vi "Update Filter.vi"(8 "error in (no error)":errorcluster, 10 "Filter in":refnum<class "Filter.lvclass">, 11 "Debugger in":refnum<class "Debugger.lvclass">) -> (0 "error out":errorcluster, 3 "Debugger out":refnum<class "Debugger.lvclass">)   [LabVIEW 2020, in "Debugger.lvclass"]
uses:
  Debugger.lvclass
  Filter/Filter.lvclass
  Debugger.lvclass/Debugger.ctl
  Debug Log/Debug Log.lvclass
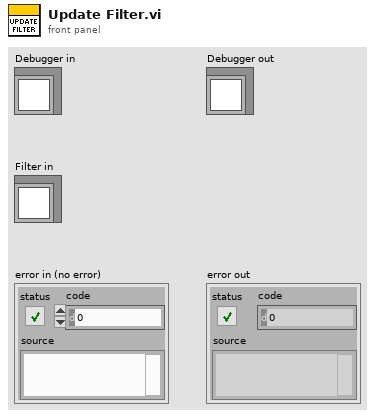
[diagram p1: front panel]
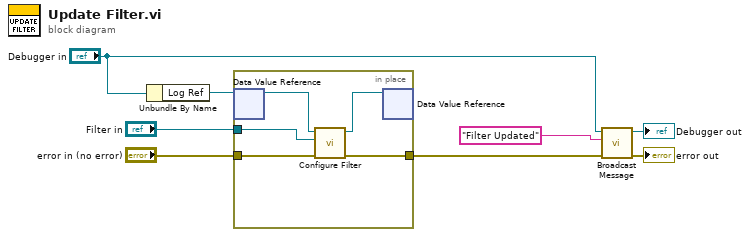
[diagram p0: block diagram]
diagram:
  n1 = Unbundle By Name("Debugger in") -> ("Log Ref"=w1:refnum<data-value>)
  n2 = in-place {
    in-place-border: "error in (no error)" -> [w13]
    in-place-border: "Filter in" -> [w12]
    in-place-border: [w11] -> w6
    n3 = in-place-dvr #1(w1) -> (w10:refnum<class "Debug Log.lvclass">)  [unwired: 1 out]
    n4 = call "Configure Filter.vi"("error in (no error)"=w13, "Filter"=w12, "Debug Log In"=w10) -> ("error out"=w11:errorcluster, "Debug Log Out"=w9:refnum<class "Debug Log.lvclass">)  [unwired: 7 in]
    n5 = in-place-dvr #1(w9) -> ()  [unwired: 2 out]
  }
  n6 = call-dynamic "Broadcast Message.vi"("error in (no error)"=w6, "Message"="Filter Updated", "Process In"="Debugger in") -> ("error out"=→"error out":errorcluster, "Process Out"=→"Debugger out":refnum<class "Debugger.lvclass">)  [unwired: 7 in]
